vi "TDT-Write DO.vi"(0 "RPcox":refnum<k7>, 5 "Next Buffer":i32, 7 "Input array":bool[][](array[boolean]), 9 "Chans":i32[](array[numeric]), 11 "error in (no error)":errorcluster) -> (4 "RPcox (thru)":refnum<k7>, 15 "error out":errorcluster)   [LabVIEW 2020]
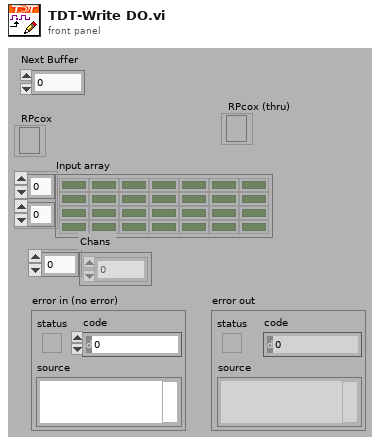
[diagram p1: front panel]
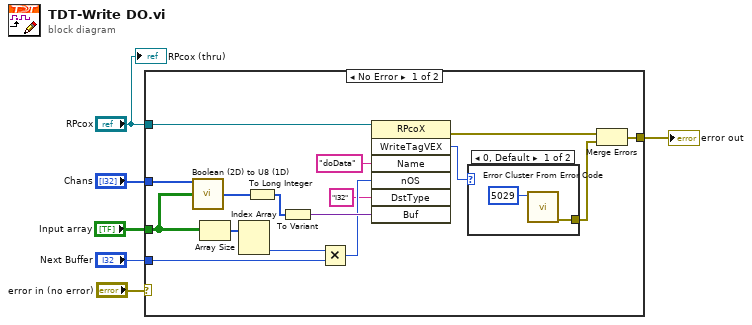
[diagram p0: block diagram]
diagram:
  n1 = case shown="No Error" "error in (no error)" {
    selector: "error in (no error)" -> [_ w25]
    tunnel: "Next Buffer" -> [w22 _]
    tunnel: "Input array" -> [w8 _]
    tunnel: "RPcox" -> [w21 _]
    tunnel: [w20 w25] -> w2
    tunnel: "Chans" -> [w9 _]
    frame No Error {
      n2 = call "Boolean (2D) to U8 (1D).vi"("Bits"=w9, "Data"=w8) -> ("sum"=w7:u8[])  [unwired: 13 in]
      n3 = Array Size(array=w8) -> (size(s)=w12:i32[])
      n4 = Index Array(array=w12) -> (element #2=w10:i32)  [unwired: 2 in, 1 out]
      n5 = To Long Integer(number=w7) -> (32bit integer=w11:i32[])
      n6 = To Variant(anything=w11) -> (Variant=w18:variant)
      n7 = Multiply(x=w10, y=w22) -> (x*y=w17:i32)
      n8 = invoke class="RPcoX" method="WriteTagVEX"(reference=w21, "Name"="doData", "nOS"=w17, "DstType"="I32", "Buf"=w18) -> (error out=w19:errorcluster, "WriteTagVEX"=w15:i32)  [unwired: 2 in, 5 out]
      n9 = case shown="0, Default" w15 {
        tunnel: [w23 _] -> w14
        frame 0, Default {
          n10 = call <vilib>:"Error Cluster From Error Code.vi"("error code (0)"=5029) -> ("error out"=w23:errorcluster)  [unwired: 8 in]
        }
        frame 1 {
        }
      }
      n11 = Merge Errors(w19, w14) -> (w20:errorcluster)
    }
    frame Error {
    }
  }
  "error out" <- w2
  "RPcox (thru)" <- "RPcox"
